vi "Read Parity.vi"(8 "error in (no error)":errorcluster, 11 "Serial Master in":refnum<class "Serial Master.lvclass">) -> (0 "error out":errorcluster, 2 "Parity":u16(ring) items=["None", "Odd", "Even", "Mark", "Space"], 3 "Serial Master out":refnum<class "Serial Master.lvclass">)   [LabVIEW 2021, in "Serial Master.lvclass"]
uses:
  Serial Master.lvclass
  Serial Master.lvclass/Serial Master.ctl
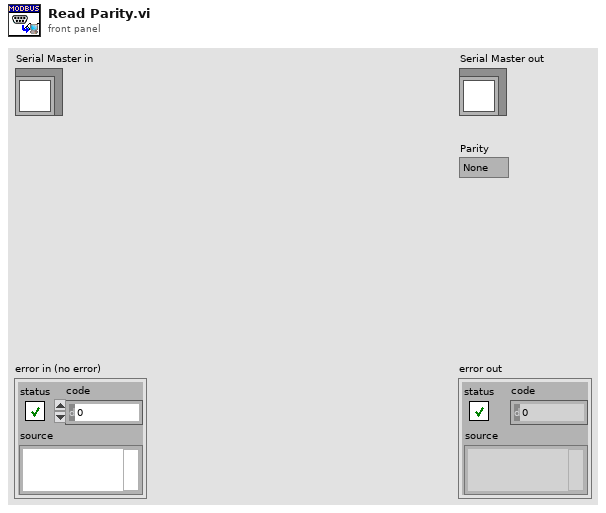
[diagram p1: front panel]
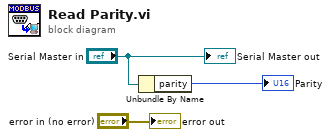
[diagram p0: block diagram]
diagram:
  n1 = Unbundle By Name("Serial Master in") -> ("parity"=→"Parity":enum16{"None", "Odd", "Even", "Mark", "Space"})
  "error out" <- "error in (no error)"
  "Serial Master out" <- "Serial Master in"
